vi "DAQmx Physical Channel Name.vi"(1 "DAQmx Physical Channel Name":tag) -> (0 "DAQmx Physical Channel Name Out":tag)   [LabVIEW 2010]
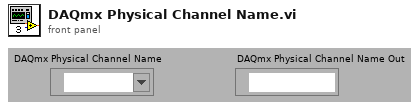
[diagram p1: front panel]
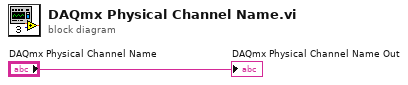
[diagram p0: block diagram]
diagram:
  "DAQmx Physical Channel Name Out" <- "DAQmx Physical Channel Name"
